vi "Teardown.vi"(8 "error in (no error)":errorcluster, 11 "LUnit Test Case In":refnum<class "LUnit Test Case.lvclass">) -> (0 "error out":errorcluster, 3 "LUnit Test Case Out":refnum<class "LUnit Test Case.lvclass">)   [LabVIEW 2020, in "LUnit Test Case.lvclass"]
doc: "Teardown method called by the testing framework to tear down test fixture after each test method is called."
uses:
  LUnit Test Case.lvclass
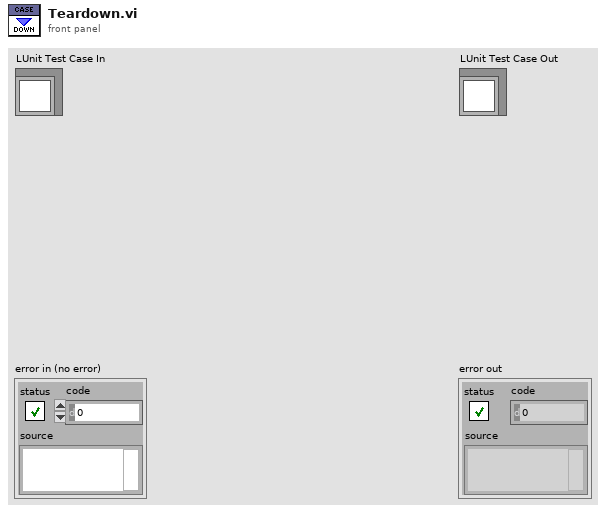
[diagram p1: front panel]
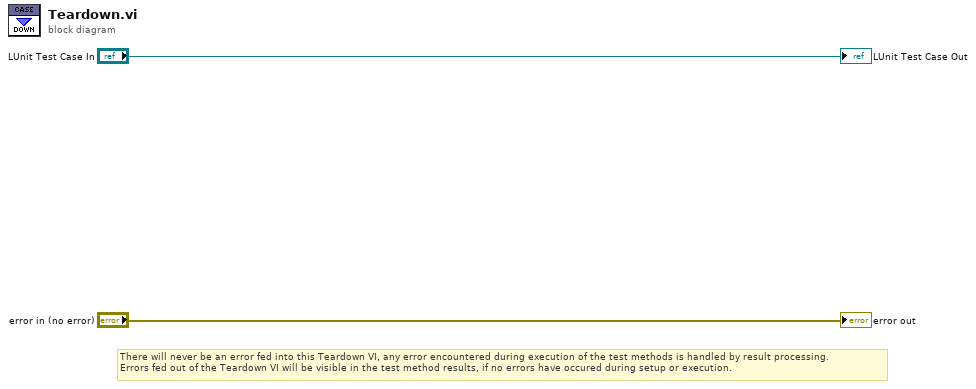
[diagram p0: block diagram]
diagram:
  # "There will never be an error fed into this Teardown VI, any error encountered during execution of the test methods is handled by result processing.\nErrors fed out of the Teardown VI will be visible in the test method results, if no errors have occured during setup or execution."
  "error out" <- "error in (no error)"
  "LUnit Test Case Out" <- "LUnit Test Case In"
